vi "Remove_duplicates(1d string).vi"(11 "In":string[](array[string])=["A", "A", "A"]) -> (3 "Out":string[](array[string]))   [LabVIEW 2017]
doc: "Use this VI to remove duplicate, adjacent elements from an array. To use this VI, enter values in the \"In\" array and run."
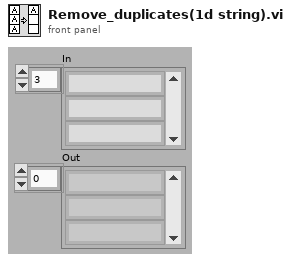
[diagram p1: front panel]
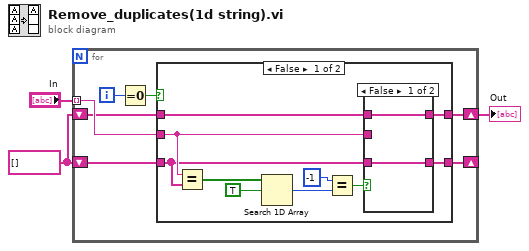
[diagram p0: block diagram]
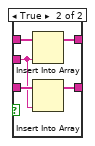
[diagram p2: hidden frame]
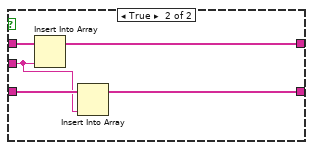
[diagram p3: hidden frame]
diagram:
  w1 = string[] []
  n1 = for {
    tunnel: "In" -> [w8] mode=indexing
    shift-right: [w6] -> _
    shift-left: w1 -> [w5]
    shift-right: [w7] -> w3
    shift-left: w1 -> [w4]
    i -> [w10]
    n2 = Equal To 0?(x=w10) -> (x = 0?=w9:bool)
    n3 = case shown="False" w9 {
      tunnel: w8 -> [w17 w28]
      tunnel: [w18 w31] -> w7
      tunnel: [w20 w29] -> w6
      tunnel: w5 -> [w16 w30]
      tunnel: w4 -> [w19 w32]
      frame False {
        n4 = Equal?(x=w17, y=w16) -> (x = y?=w15:bool[])
        n5 = Search 1D Array(1D array=w15, element=TRUE ("盔家")) -> (index of element=w13:i32)  [unwired: 1 in]
        n6 = Equal?(x=-1, y=w13) -> (x = y?=w11:bool)
        n7 = case shown="False" w11 {
          tunnel: w16 -> [w22 w25]
          tunnel: [w22 w24] -> w20
          tunnel: [w21 w26] -> w18
          tunnel: w19 -> [w21 w27]
          tunnel: w17 -> [_ w23]
          frame False {
          }
          frame True {
            n8 = Insert Into Array(array=w27, new element=w23) -> (w26:string[])  [unwired: 1 in]
            n9 = Insert Into Array(array=w25, new element=w23) -> (w24:string[])  [unwired: 1 in]
          }
        }
      }
      frame True {
        n10 = Insert Into Array(array=w32, new element=w28) -> (w31:string[])  [unwired: 1 in]
        n11 = Insert Into Array(array=w30, new element=w28) -> (w29:string[])  [unwired: 1 in]
      }
    }
  }
  "Out" <- w3
